vi "Agilent 4263X Multiple Measurements.vi"() -> ()   [LabVIEW 2016]
doc: "This Example VI configures the instrument to take a specified number of measurements of the selected primary and secondary functions.\n\nThe bus trigger (:TRIG) is used to trigger measurements which are then fed to the data buffers which are then read.\n\nThe instrument should be first initialized with the Initialize VI (ID query and Reset should be set to yes).\n\nThis VI sets the primary and secondary measurement types along with the trigger mode (bus), averaging rate, and number of data points. The VI then reads the primary and secondary data buffers."
uses:
  <instrlib>/Agilent 4263X/Agilent 4263X.lvlib
panel:
  in  "VISA resource name":refnum<visa-resource-name>
  in  "averaging count (1)":i16=1 min=1 max=256 step=1
  out "secondary data":T1(array[cluster]) {"data" format="%.5e"}
  out "primary data":T1(array[cluster]) {"data" format="%.5e"}
  in  "number of data points (10)":i16=10 min=1 max=200 step=1
  in  "function (Z - Angle:0)":u16(ring) items=["Z - Angle", "R - X", "Y - Angle", "G - B", "CP - D", "CP - Q", "CP - G", "CS - D", "CS - Q", "CS - RS", "LP - D", "LP - Q", "LP - G", "LS - D", "LS - Q", "LS - RS", "LS - DCR (option 001 only)", "LP - DCR (option 001 only)", "L2 - N (option 001 only)", "L2 - M (option 001 only)", "L2 - R2 (option 001 only)"]
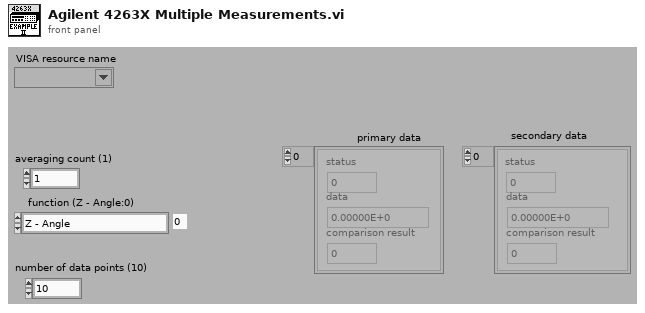
[diagram p1: front panel]
types:
  T1 = cluster{"status":u16, "data":dbl, "comparison result":u16}[]
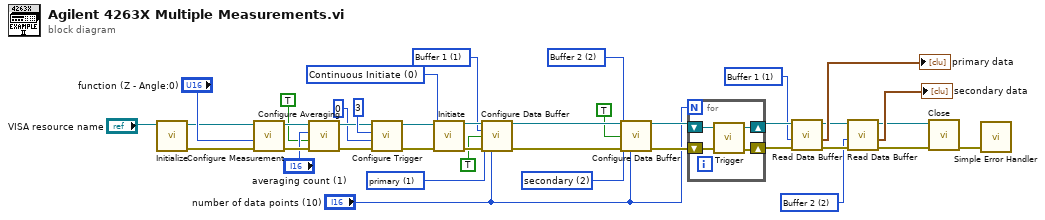
[diagram p0: block diagram]
diagram:
  w2 = u16 2 items=["Buffer 1"=1, "Buffer 2"=2] ("buffer (1:buffer 1)")
  w3 = u16 1 items=["Buffer 1"=1, "Buffer 2"=2] ("buffer (1:buffer 1)")
  w4 = u16 2 items=["primary"=1, "secondary"=2] ("function (1:primary)")
  w5 = u16 2 items=["Buffer 1"=1, "Buffer 2"=2] ("buffer (1:Buffer 1)")
  w7 = u16 1 items=["primary"=1, "secondary"=2] ("function (1:primary)")
  w8 = u16 1 items=["Buffer 1"=1, "Buffer 2"=2] ("buffer (1:Buffer 1)")
  w10 = u16 0 items=["Continuous Initiate", "Single Initiate", "Stop Continuous"] ("initiate mode (0:continuous)")
  n1 = call <instrlib>:"Initialize.vi"("VISA resource name"="VISA resource name") -> ("error out"=w11:errorcluster, "VISA resource name out"=w12:refnum<visa-resource-name>)  [unwired: 9 in]
  n2 = call <instrlib>:"Configure Measurement.vi"("error in (no error)"=w11, "function (Z - Angle:0)"="function (Z - Angle:0)", "VISA resource name"=w12) -> ("error out"=w18:errorcluster, "VISA resource name out"=w21:refnum<visa-resource-name>)  [unwired: 7 in]
  n3 = call <instrlib>:"Configure Averaging.vi"("error in (no error)"=w18, "Enable Averge Mode  (on:T)"=TRUE, "Average count (1)"="averaging count (1)", "VISA resource name"=w21) -> ("error out"=w19:errorcluster, "VISA resource name out"=w20:refnum<visa-resource-name>)  [unwired: 6 in]
  n4 = call <instrlib>:"Configure Trigger.vi"("error in (no error)"=w19, "trigger delay (sec)"=0, "trigger source (int:0)"=3, "VISA resource name"=w20) -> ("error out"=w39:errorcluster, "VISA resource name out"=w38:refnum<visa-resource-name>)  [unwired: 6 in]
  n5 = call <instrlib>:"Initiate.vi"("error in (no error)"=w39, "initiate mode (0:continuous)"=w10, "VISA resource name"=w38) -> ("error out"=w35:errorcluster, "VISA resource name out"=w34:refnum<visa-resource-name>)  [unwired: 7 in]
  n6 = call <instrlib>:"Configure Data Buffer.vi"("VISA resource name"=w34, "buffer (1:Buffer 1)"=w8, "Enable buffer feed (T)"=TRUE, "function (1:primary)"=w7, "error in (no error)"=w35, "number of points (10)"="number of data points (10)") -> ("VISA resource name out"=w31:refnum<visa-resource-name>, "error out"=w32:errorcluster)  [unwired: 8 in]
  n7 = call <instrlib>:"Configure Data Buffer.vi"("VISA resource name"=w31, "buffer (1:Buffer 1)"=w5, "Enable buffer feed (T)"=TRUE, "function (1:primary)"=w4, "error in (no error)"=w32, "number of points (10)"="number of data points (10)") -> ("VISA resource name out"=w25:refnum<visa-resource-name>, "error out"=w26:errorcluster)  [unwired: 8 in]
  n8 = for {
    N: "number of data points (10)" -> [_]
    shift-right: [w42] -> w22
    shift-left: w26 -> [w43]
    shift-right: [w41] -> w23
    shift-left: w25 -> [w40]
    n9 = call <instrlib>:"Trigger.vi"("error in (no error)"=w43, "VISA resource name"=w40) -> ("error out"=w42:errorcluster, "VISA resource name out"=w41:refnum<visa-resource-name>)  [unwired: 8 in]
  }
  n10 = call <instrlib>:"Read Data Buffer.vi"("error in (no error)"=w22, "buffer (1:buffer 1)"=w3, "VISA resource name"=w23) -> ("error out"=w28:errorcluster, "data buffer"=→"primary data":T1, "VISA resource name out"=w29:refnum<visa-resource-name>)  [unwired: 6 in]
  n11 = call <instrlib>:"Read Data Buffer.vi"("error in (no error)"=w28, "buffer (1:buffer 1)"=w2, "VISA resource name"=w29) -> ("error out"=w14:errorcluster, "data buffer"=→"secondary data":T1, "VISA resource name out"=w15:refnum<visa-resource-name>)  [unwired: 6 in]
  n12 = call <instrlib>:"Close.vi"("error in (no error)"=w14, "VISA resource name"=w15) -> ("error out"=w1:errorcluster)  [unwired: 9 in]
  n13 = call <vilib>:"Simple Error Handler.vi"("error in (no error)"=w1) -> ()  [unwired: 4 in, 5 out]
